vi "Read Max Min Waveform.vi"(8 "error in (no error)":errorcluster, 9 "Timeout (10000 ms)":u32=10000, 10 "Source (0: Channel 1)":u16(ring) items=["Channel 1", "Channel 2", "Channel 3", "Channel 4", "Memory 1", "Memory 2", "Memory 3", "Memory 4", "Function 1", "Function 2", "Function 3", "Function 4", "Function 5", "Function 6", "Function 7", "Function 8"], 11 "VISA resource name":refnum<visa-resource-name>) -> (0 "error out":errorcluster, 1 "Min Waveform":waveform(dbl)(graph), 2 "Max Waveform":waveform(dbl)(graph), 3 "VISA resource name out":refnum<visa-resource-name>)   [LabVIEW 2018, in "LeCroy Wave Series.lvlib"]
doc: "Returns the two waveforms the oscilloscope acquired for the specified channel. The waveforms are from an acquisition that you initiate prior to calling this VI. A both waveforms must be in one channel together. It is usable for math functions, for example math function envelope get two waveforms. One is roof and second is floor."
uses:
  LeCroy Wave Series.lvlib
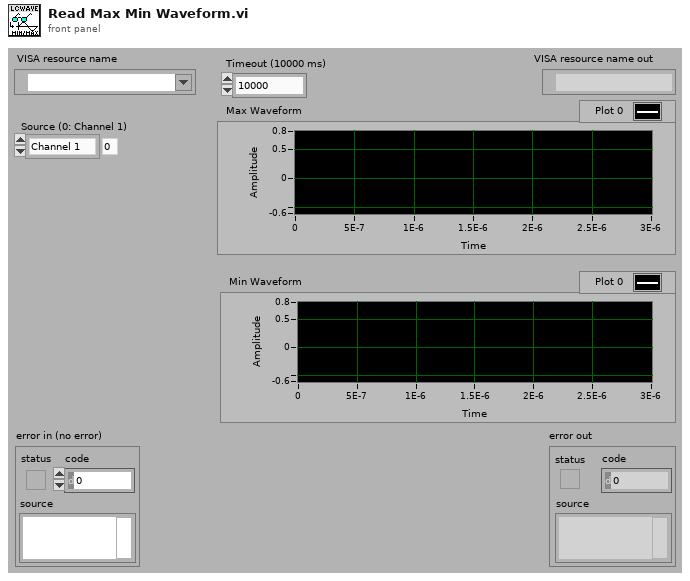
[diagram p1: front panel]
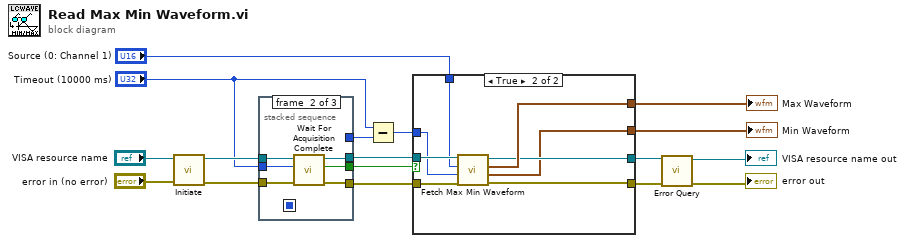
[diagram p0: block diagram]
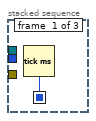
[diagram p2: hidden frame]
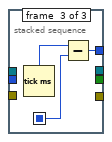
[diagram p3: hidden frame]
diagram:
  n1 = call "Initiate.vi"("error in (no error)"="error in (no error)", "VISA resource name"="VISA resource name") -> ("error out"=w12:errorcluster, "VISA resource name out"=w13:refnum<visa-resource-name>)  [unwired: 8 in]
  n2 = stacked-sequence {
    seq-local: [w18 _ _] -> [_ _ w26]
    tunnel: "Timeout (10000 ms)" -> [_ w24 _]
    tunnel: w13 -> [_ w22 _]
    tunnel: w12 -> [_ w20 _]
    tunnel: [_ w19 _] -> w10
    tunnel: [_ w21 _] -> w11
    tunnel: [_ _ w25] -> w8
    tunnel: [_ w23 _] -> w6
    frame #0 {
      n3 = Tick Count (ms)() -> (millisecond timer value=w18:u32)
    }
    frame #1 {
      n4 = call "Wait For Acquisition Complete.vi"("error in (no error)"=w20, "Timeout (10000 ms)"=w24, "VISA resource name"=w22) -> ("error out"=w19:errorcluster, "Complete"=w23:bool, "VISA resource name out"=w21:refnum<visa-resource-name>)  [unwired: 6 in]
    }
    frame #2 {
      n5 = Tick Count (ms)() -> (millisecond timer value=w27:u32)
      n6 = Subtract(x=w27, y=w26) -> (x-y=w25:u32)
    }
  }
  n7 = Subtract(x="Timeout (10000 ms)", y=w8) -> (x-y=w7:u32)
  n8 = case shown="True" w6 {
    tunnel: w11 -> [w29 w37]
    tunnel: w10 -> [w28 w36]
    tunnel: "Source (0: Channel 1)" -> [_ w35]
    tunnel: [_ w34] -> w14
    tunnel: [w29 w33] -> w5
    tunnel: [w28 w32] -> w3
    tunnel: w7 -> [_ w31]
    tunnel: [_ w30] -> w1
    frame False {
    }
    frame True {
      n9 = call "Fetch Max Min Waveform.vi"("error in (no error)"=w36, "Timeout (10000 ms)"=w31, "Source (0: Channel 1)"=w35, "VISA resource name"=w37) -> ("error out"=w32:errorcluster, "Min"=w30:waveform(dbl), "Max"=w34:waveform(dbl), "VISA resource name out"=w33:refnum<visa-resource-name>)  [unwired: 4 in]
    }
  }
  "Max Waveform" <- w14
  "Min Waveform" <- w1
  n10 = call "Error Query.vi"("error in (no error)"=w3, "VISA resource name"=w5) -> ("error out"=→"error out":errorcluster, "VISA resource name out"=→"VISA resource name out":refnum<visa-resource-name>)  [unwired: 6 in, 2 out]
